vi "Do.vi"(8 "error in (no error)":errorcluster, 10 "Actor in":refnum<class "Actor.lvclass">, 11 "Write All Pulse Msg":refnum<class "Write All Pulse Msg.lvclass">) -> (0 "error out":errorcluster, 2 "Actor out":refnum<class "Actor.lvclass">)   [LabVIEW 2019, in "Electronic Load.lvlib" / "Write All Pulse Msg.lvclass"]
doc: "This VI delivers the message to the actor by calling the appropriate method(s) on the actor."
uses:
  Write All Pulse Msg.lvclass
  builds/Engine/Actor Framework.lvlibp/1abvi3w/vi.lib/ActorFramework/Actor/Actor.lvclass
  Library/Electronic Load.lvclass
  C:/Users/Public/Documents/Development/builds/Engine/Actor Framework.lvlibp/1abvi3w/vi.lib/ActorFramework/Actor/Actor.lvclass
  Write All Pulse Msg.lvclass/Write All Pulse Msg.ctl
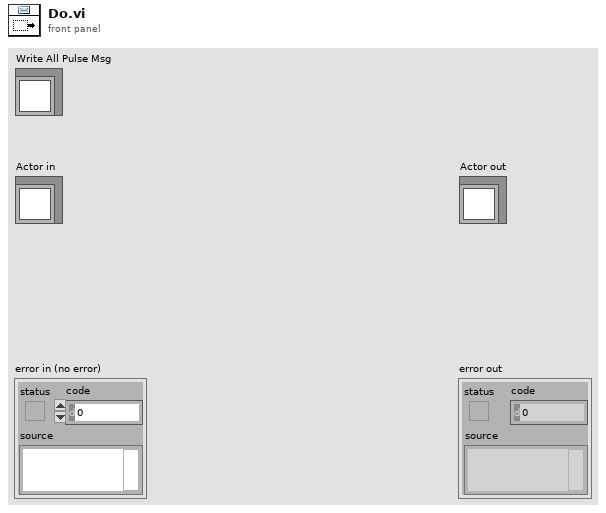
[diagram p1: front panel]
types:
  T1 = typedef "Electronic Load.lvlib/Electronic Load.lvclass/Trigger Settings.ctl" = cluster{"Mode":T2, "Initial":dbl, "Transient":dbl, "Interval":dbl, "Width":dbl, "Delay":dbl, "Data Pts":i32, "Slew Rate":dbl}
  T2 = typedef "Electronic Load.lvlib/Electronic Load.lvclass/E-Load Mode.ctl" = enum16{"Current", "Resistance", "Voltage"}
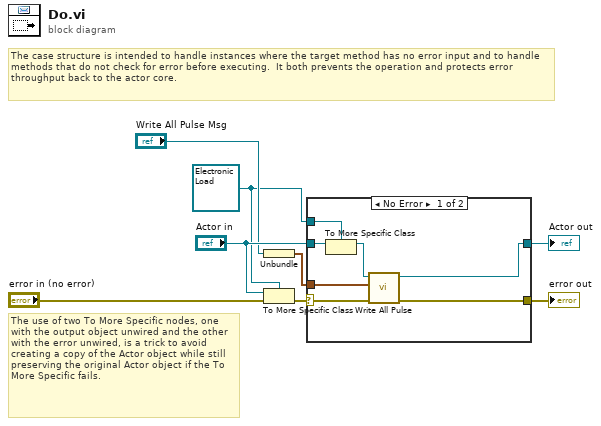
[diagram p0: block diagram]
diagram:
  w3 = refnum<class "Electronic Load.lvclass"> refnum ("Actor in")
  # "The use of two To More Specific nodes, one with the output object unwired and the other with the error unwired, is a trick to avoid creating a copy of the Actor object while still preserving the original Actor object if the To More Specific fails."
  # "The case structure is intended to handle instances where the target method has no error input and to handle methods that do not check for error before executing.  It both prevents the operation and protects error throughput back to the actor core."
  n1 = Unbundle("Write All Pulse Msg") -> (w1:T1)
  n2 = To More Specific Class(target class=w3, reference="Actor in", error in="error in (no error)") -> (error out=w2:errorcluster)  [unwired: 1 out]
  n3 = case shown="No Error" w2 {
    selector: w2 -> [w13 w17]
    tunnel: [w15 w17] -> w8
    tunnel: [w14 w16] -> w7
    tunnel: "Actor in" -> [w12 w16]
    tunnel: w3 -> [w11 _]
    tunnel: w1 -> [w9 _]
    frame No Error {
      n4 = To More Specific Class(target class=w11, reference=w12) -> (specific class reference=w10:refnum<class "Electronic Load.lvclass">)  [unwired: 1 in, 1 out]
      n5 = call "Write All Pulse.vi"("error in"=w13, "Trigger Settings All"=w9, "Electronic Load in"=w10) -> ("error out"=w15:errorcluster, "Electronic Load out"=w14:refnum<class "Electronic Load.lvclass">)  [unwired: 7 in]
    }
    frame Error {
      # "If type check fails, pass the original object out again."
    }
  }
  "error out" <- w8
  "Actor out" <- w7
